vi "Update Data.vi"(8 "error in (no error)":errorcluster, 10 "Debug Data":refnum<class "Debug Data.lvclass">[](array[class]), 11 "List Seen Processes View Model In":refnum<class "List Box View Model.lvclass">) -> (0 "error out":errorcluster, 3 "List Seen Processes View Model Out":refnum<class "List Box View Model.lvclass">)   [LabVIEW 2020, in "List Box View Model.lvclass"]
uses:
  List Box View Model.lvclass
  Debug Data/Debug Data.lvclass
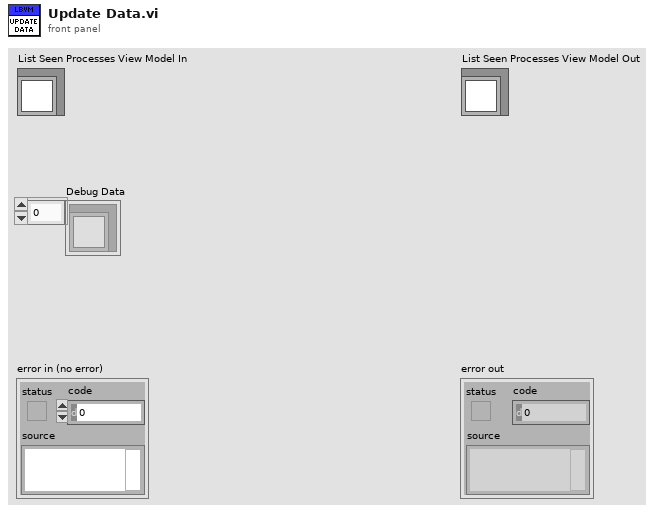
[diagram p1: front panel]
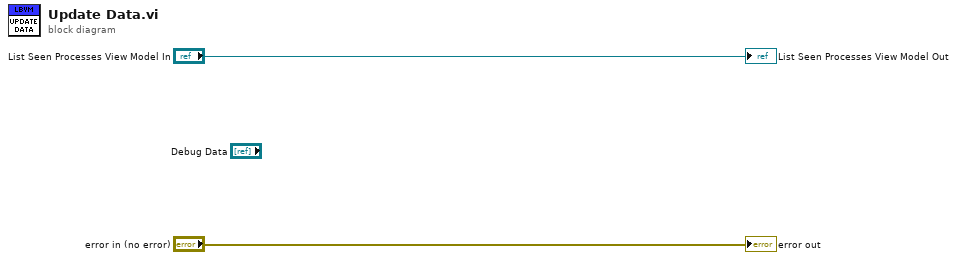
[diagram p0: block diagram]
diagram:
  "error out" <- "error in (no error)"
  "List Seen Processes View Model Out" <- "List Seen Processes View Model In"
